vi "LCDSetCharacterBitmap.vi"(7 "Font":u16(ring)=4 items=["FONT_User1"=1, "FONT_User2"=2, "FONT_6x10"=3, "FONT_5x8"=4, "FONT_6x12"=5], 8 "error in (no error)":errorcluster, 9 "Bitmap":u8[](array[numeric]), 10 "Character":string, 11 "Device In":u64) -> (0 "error out":errorcluster, 3 "Device Out":u64)   [LabVIEW 2012, in "Phidget LCD.lvlib"]
doc: "${SetCharacterBitmap:Header}"
uses:
  <instrlib>/Phidgets/Phidget LCD/Phidget LCD.lvlib
  <instrlib>/Phidgets/Phidget Common/Phidget Common.lvlib
  phidget22.dll
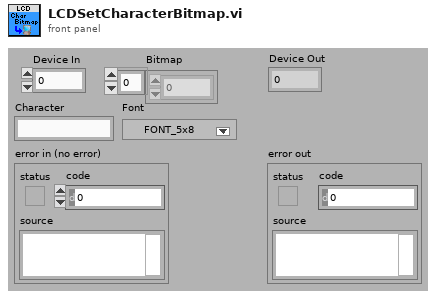
[diagram p1: front panel]
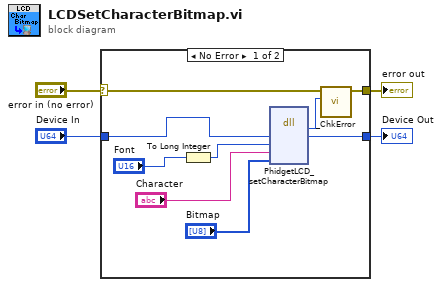
[diagram p0: block diagram]
diagram:
  n1 = case shown="No Error" "error in (no error)" {
    selector: "error in (no error)" -> [w11 w15]
    tunnel: [w10 w15] -> w3
    tunnel: "Device In" -> [w13 w14]
    tunnel: [w12 w14] -> w1
    frame No Error {
      n2 = To Long Integer(number="Font") -> (32bit integer=w8:i32)
      n3 = dll-call lib="phidget22.*" fn="PhidgetLCD_setCharacterBitmap"("phid"=w13, "font"=w8, "character"="Character", "bitmap"="Bitmap") -> ("return type"=w9:i32, "phid"=w12:u64)  [unwired: 6 in, 2 out]
      n4 = call <instrlib>:"_ChkError.vi"("Return Code"=w9, "error in (no error)"=w11) -> ("error out"=w10:errorcluster)  [unwired: 9 in]
    }
    frame Error {
    }
  }
  "error out" <- w3
  "Device Out" <- w1
